vi "Save Machine Configuration.vi"(4 "error in (no error)":errorcluster, 6 "Plugin Name":T3, 7 "TC Parameters":T2) -> (0 "error out":errorcluster, 1 "Result":T1, 2 "Changed?":bool, 3 "Plugin Name out":T3)   [LabVIEW 2015, in "Config Data.lvlib" / "Config Data.lvclass"]
uses:
  Config Data.lvclass
  Startup Processes/_typedefs/Subpanel Names.ctl
  Startup Processes/_typedefs/TC Setup Parameters.ctl
  Startup Processes/_typedefs/Pass Fail Flag.ctl
  Startup Processes/Startup Processes.lvlib
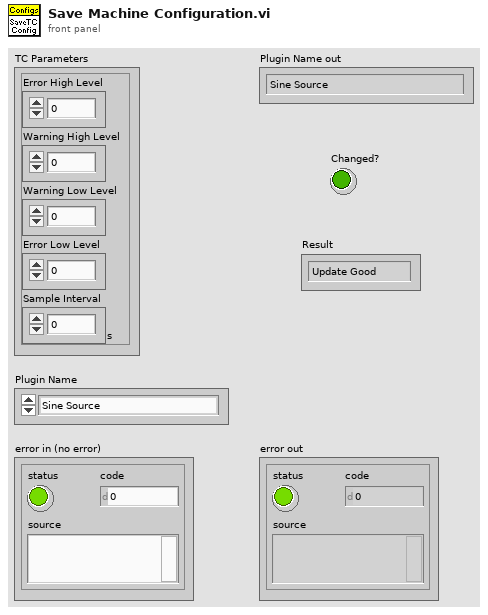
[diagram p1: front panel]
types:
  T1 = typedef "Startup Processes.lvlib/Pass Fail Flag.ctl" = enum16{"Update Good", "Update Failed"}
  T2 = typedef "Startup Processes.lvlib/TC Setup Parameters.ctl" = cluster{"Error High Level":dbl, "Warning High Level":dbl, "Warning Low Level":dbl, "Error Low Level":dbl, "Sample Interval":dbl[unit]}
  T3 = typedef "Startup Processes.lvlib/Subpanel Names.ctl" = enum16{"Sine Source", "Ramp Source", "Hen House TC", "Dog House TC", "Out House TC"}
  T4 = typedef "Startup Processes.lvlib/Data Valid Flag.ctl" = enum16{"Data Valid", "Data Not Valid"}
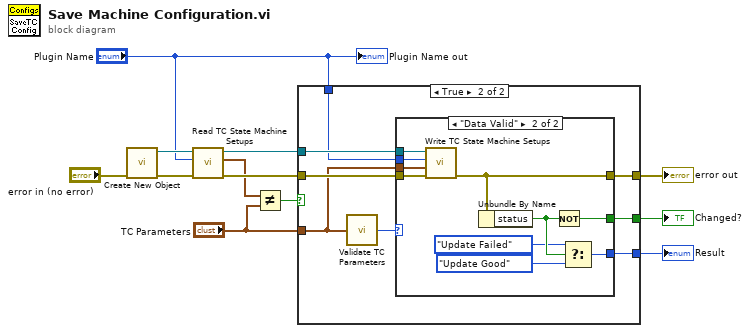
[diagram p0: block diagram]
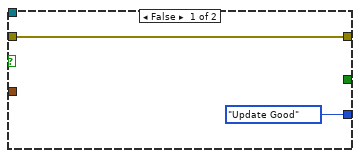
[diagram p2: hidden frame]
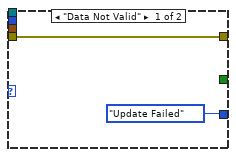
[diagram p3: hidden frame]
diagram:
  n1 = call "Create New Object.vi"("Error In"="error in (no error)") -> ("Error Out"=w10:errorcluster, "Config Data"=w9:refnum<class "Config Data.lvclass">)  [unwired: 5 in]
  n2 = call-dynamic "Read TC State Machine Setups.vi"("Error In"=w10, "Instance Name"="Plugin Name", "Config Data in"=w9) -> ("Error Out"=w7:errorcluster, "TC Parameters"=w4:T2, "Config Data out"=w8:refnum<class "Config Data.lvclass">)  [unwired: 2 in]
  n3 = Not Equal?(x=w4, y="TC Parameters") -> (x != y?=w3:bool)
  n4 = case shown="True" w3 {
    tunnel: [w14 w19] -> w11
    tunnel: w8 -> [_ w22]
    tunnel: w7 -> [w14 w21]
    tunnel: "Plugin Name" -> [_ w20]
    tunnel: "TC Parameters" -> [_ w16]
    tunnel: [_ w18] -> w2
    tunnel: [Pass_Fail_Flag."Update Good" ("f") w17] -> w1
    frame False {
    }
    frame True {
      n5 = call "Validate TC Parameters.vi"("TC Parameters"=w16) -> ("Result"=w15:T4)
      n6 = case shown="\"Data Valid\"" w15 {
        tunnel: w22 -> [_ w34]
        tunnel: w21 -> [w24 w33]
        tunnel: w20 -> [_ w32]
        tunnel: [w24 w31] -> w19
        tunnel: [_ w30] -> w18
        tunnel: [Pass_Fail_Flag."Update Failed" ("f") w28] -> w17
        tunnel: w16 -> [_ w26]
        frame "Data Not Valid" {
        }
        frame "Data Valid" {
          n7 = call-dynamic "Write TC State Machine Setups.vi"("Error In"=w33, "TC Parameters"=w26, "Instance Name"=w32, "Config Data in"=w34) -> ("Error Out"=w31:errorcluster)  [unwired: 2 in, 1 out]
          n8 = Unbundle By Name(w31) -> ("status"=w29:bool)
          n9 = Not(x=w29) -> (.not. x?=w30:bool)
          n10 = Select(t=Pass_Fail_Flag."Update Failed" ("Result"), s=w29, f=Pass_Fail_Flag."Update Good") -> (s? t:f=w28:T1)
        }
      }
    }
  }
  "error out" <- w11
  "Changed?" <- w2
  "Result" <- w1
  "Plugin Name out" <- "Plugin Name"
